vi "RefreshSubTree.vi"(8 "error in":errorcluster, 10 "node information":T1[](array[typedef]), 11 "tree ref in":refnum<vi>) -> (0 "error out":errorcluster, 3 "tree ref out":refnum<vi>)   [LabVIEW 2013, in "NISE_CEF_TreeControl.lvlib"]
doc: "Updates just a portion of the tree control"
uses:
  NISE_CEF_TreeControl.lvlib
  Node/Summary.ctl
  Node/NISE_CEF_Node.lvclass
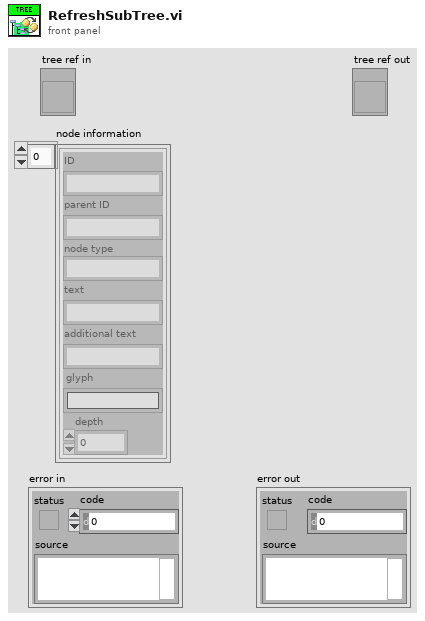
[diagram p1: front panel]
types:
  T1 = typedef "NISE_CEF_Node.lvclass/Summary.ctl" = cluster{"ID":string, "parent ID":string, "node type":string, "text":string, "additional text":string, "glyph":string, "depth":i32}
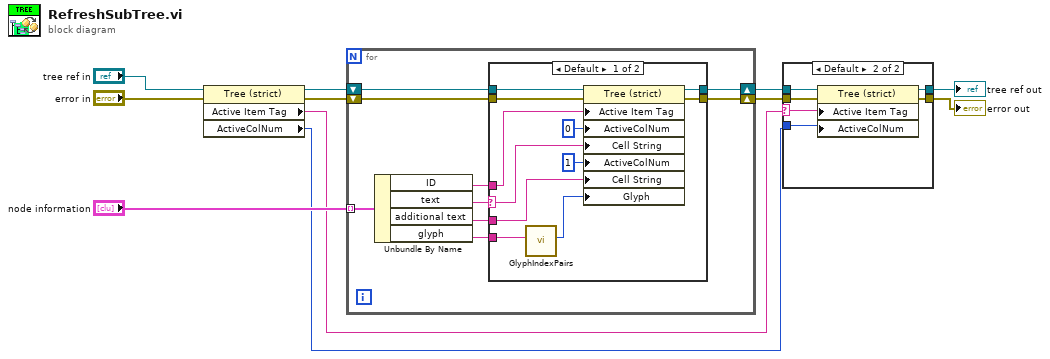
[diagram p0: block diagram]
diagram:
  n1 = property class="Tree (strict)"(reference="tree ref in", error in="error in") -> (reference out=w9:refnum<vi>, error out=w7:errorcluster, "Active Item Tag"=w2:string, "ActiveColNum"=w1:i32)
  n2 = for {
    shift-right: [w19] -> w3
    shift-left: w7 -> [w18]
    tunnel: "node information" -> [w20] mode=indexing
    shift-right: [w16] -> w4
    shift-left: w9 -> [w15]
    n3 = Unbundle By Name(w20) -> ("ID"=w14:string, "text"=w17:string, "additional text"=w13:string, "glyph"=w12:string)
    n4 = case shown="Default" w17 {
      selector: w17 -> [w25 _]
      tunnel: [w28 w33] -> w19
      tunnel: w18 -> [w29 w33]
      tunnel: [w30 w32] -> w16
      tunnel: w15 -> [w31 w32]
      tunnel: w14 -> [w27 _]
      tunnel: w13 -> [w23 _]
      tunnel: w12 -> [w22 _]
      frame Default {
        n5 = call "GlyphIndexPairs.vi"("glyph"=w22) -> ("index"=w21:i32)  [unwired: 10 in]
        n6 = property class="Tree (strict)"(reference=w31, error in=w29, "Active Item Tag"=w27, "ActiveColNum"=0 ("Active Cell:Active Column Number"), "Cell String"=w25, "ActiveColNum"=1 ("Active Cell:Active Column Number"), "Cell String"=w23, "Glyph"=w21) -> (reference out=w30:refnum<vi>, error out=w28:errorcluster)
      }
      frame "" {
      }
    }
  }
  n7 = case shown="Default" w2 {
    selector: w2 -> [_ w36]
    tunnel: [w35 w41] -> w5
    tunnel: w4 -> [w35 w40]
    tunnel: w3 -> [w34 w39]
    tunnel: w1 -> [_ w38]
    tunnel: [w34 w37] -> w6
    frame "" {
    }
    frame Default {
      n8 = property class="Tree (strict)"(reference=w40, error in=w39, "Active Item Tag"=w36, "ActiveColNum"=w38) -> (reference out=w41:refnum<vi>, error out=w37:errorcluster)
    }
  }
  "tree ref out" <- w5
  "error out" <- w6
